vi "Read Field.vi"(7 "field name":string, 8 "error in (no error)":errorcluster, 9 "type code":T1, 10 "value":variant, 11 "Value in":refnum<class "Value.lvclass">) -> (0 "error out":errorcluster, 2 "value out":variant, 3 "Value out":refnum<class "Value.lvclass">)   [LabVIEW 2020, in "Value.lvlib" / "Value.lvclass"]
uses:
  Value.lvclass
  <vilib>/ErrorRing/Error Ring.xnode
  3e63842f-1b42-44b7-bfbc-53574ae558bd.vi
  0df52538-0c37-4fc1-a2a6-aa64d23bd73e.vi
  ea7cb730-9445-4e63-a674-7488b051f0a2.vi
  ecc6d044-d1d6-4258-b554-93b542f000c4.vi
  f0dd0353-13dc-4229-be36-72f5216b3ba3.vi
  663b7534-5be4-4c26-8693-775dffd107bf.vi
  6d95b702-a3d4-47fa-b99c-6e9c691d9abd.vi
  334379f0-c2c1-4fd4-b37a-a75153a3c3c1.vi
  22215a59-2fe5-468e-8a76-07a567f1422d.vi
  3b673ad6-c2bb-415d-ac32-dac8d0585a62.vi
  4907590c-51dd-452d-854a-3f23d6337043.vi
  91e94b60-106e-4a8f-bb72-5d9817169e6a.vi
  c7390ac7-e1e0-4f30-b90a-9159575d946d.vi
  aaf6655d-cd8e-45f8-b77e-a22837ed21e0.vi
  830d96f2-0dcb-4e12-99cb-9e6dde05f73e.vi
  77dc8c9c-6059-4e17-8748-14fb7ec0ac2f.vi
  a9875d30-4bd9-4a8c-a52c-f68dec12aa6b.vi
  6dbc08b8-92b8-4054-99f1-d97896c52856.vi
  c55a9e90-05cb-4a8a-8098-6274f5663967.vi
  316c9c8d-b543-4ebf-942d-59175514938d.vi
  229b0493-3b28-4ef3-8240-f1556a969e00.vi
  76e9d66a-8186-463b-a0b5-702645c41f9e.vi
  c324c6c0-264f-44f1-9003-e2f03347ce10.vi
  99229403-bf4d-41b1-8e34-2119cf99b534.vi
  94649a53-8ca4-4095-9f16-4726c07ca332.vi
  d57c28cb-9096-4c65-b10b-a5dea6344eea.vi
  a983453c-48a8-483e-9635-4b6015360bbf.vi
  3184ba56-7df3-4453-b731-c59013ebea68.vi
  6054442b-7a6b-42bc-83b9-383781339b04.vi
  6affac03-527b-4ec4-b0fc-9a513264455a.vi
  a9131e02-a07e-4dd8-b605-98a98183cd4d.vi
  df721e5c-d840-4c3d-88a1-754951405b27.vi
  37bd5290-b6b7-48eb-a0fa-e2d498b26fe2.vi
  1f354738-e960-4e7d-8bfb-2b975031cf57.vi
  eb45627c-0224-4171-a2ca-7d038fcf7cb5.vi
  763b9c78-21ee-42ab-85a7-a612ad3e0854.vi
  b475763c-3eeb-44d5-9789-6e92f77c8c05.vi
  7e13b756-e5dd-4f30-8145-3e48ab5751a0.vi
  311b836b-25cf-44d6-867a-da423852ab29.vi
  884a57a7-1cc5-4241-a283-3421418f3c32.vi
  e5b34253-12a8-4f36-ae48-ef8a9a19dc9f.vi
  9a6462e7-f1a7-4896-b94c-43e163632ccd.vi
  919939b4-f74b-49d6-a078-a721f5adc92b.vi
  7b5734c8-9551-4087-a43c-2e9c6be36d77.vi
  e7c0ed72-c8d2-4a6e-8d95-57b650344be6.vi
  78a636ab-c8c7-43d5-9c2f-ed25fd418a22.vi
  3f976d8e-f489-4d6c-8102-c644feb36fb3.vi
  2b071918-53f3-414b-a359-069b1376627a.vi
  60c7cc55-0a77-42d8-819b-5811e97bdf1a.vi
  <vilib>/Utility/error.llb/Error Cluster From Error Code.vi
  Type Code.ctl
  Value.lvlib
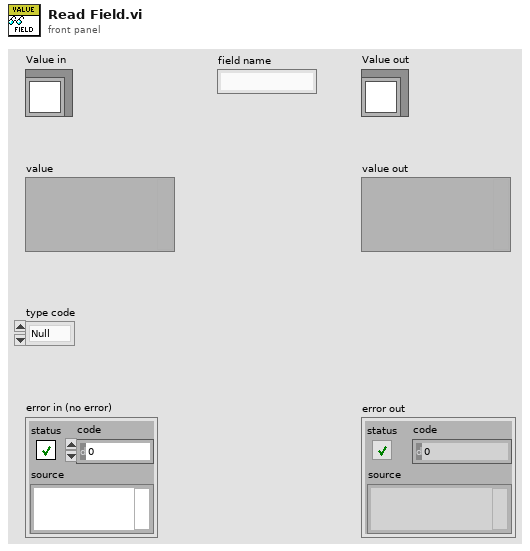
[diagram p1: front panel]
types:
  T1 = typedef "Value.lvlib/Type Code.ctl" = enum8{"Null", "Bool", "BoolA", "Int8", "Int8A", "Int16", "Int16A", "Int32", "Int32A", "Int64", "Int64A", "UInt8", "UInt8A", "UInt16", "UInt16A", "UInt32", "UInt32A", "UInt64", "UInt64A", "Float32", "Float32A", "Float64", "Float64A", "String", "StringA", "Struct", "StructA", "Union", "UnionA", "Any", "AnyA"}
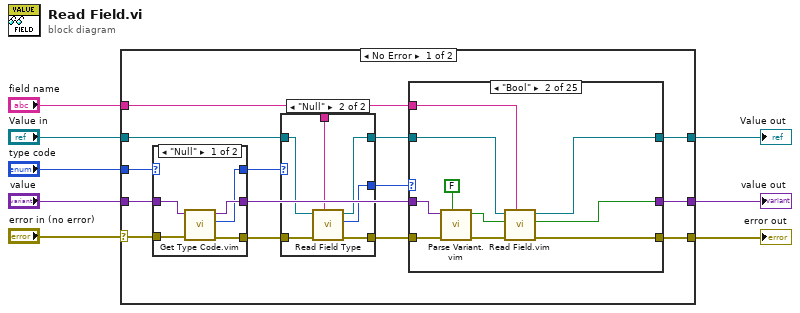
[diagram p0: block diagram]
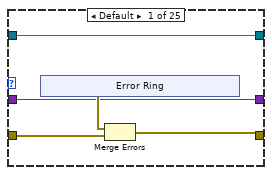
[diagram p4: hidden frame]
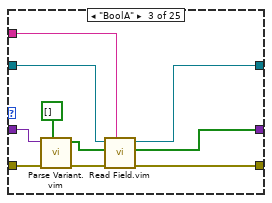
[diagram p5: hidden frame]
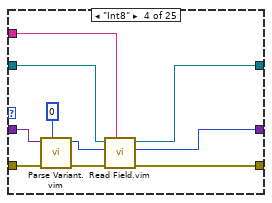
[diagram p6: hidden frame]
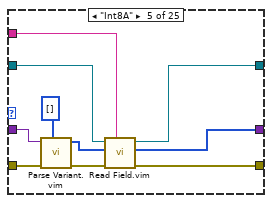
[diagram p7: hidden frame]
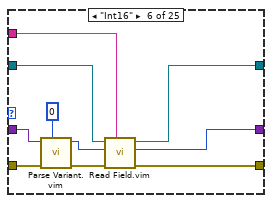
[diagram p8: hidden frame]
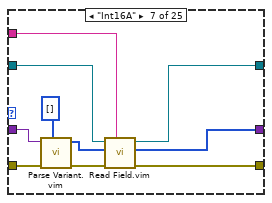
[diagram p9: hidden frame]
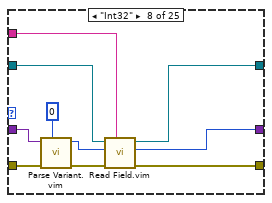
[diagram p10: hidden frame]
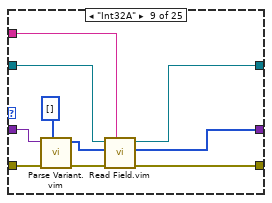
[diagram p11: hidden frame]
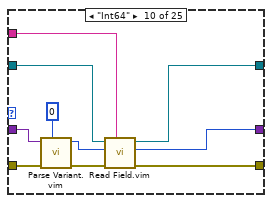
[diagram p12: hidden frame]
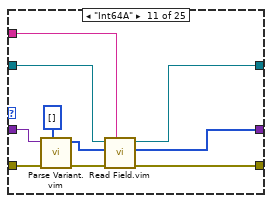
[diagram p13: hidden frame]
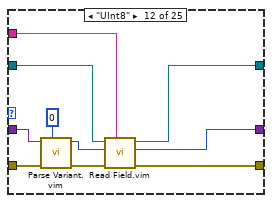
[diagram p14: hidden frame]
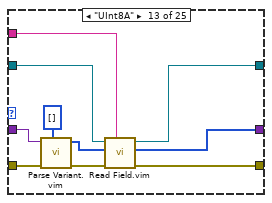
[diagram p15: hidden frame]
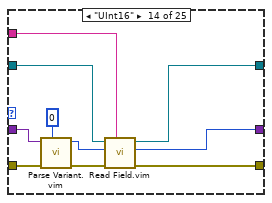
[diagram p16: hidden frame]
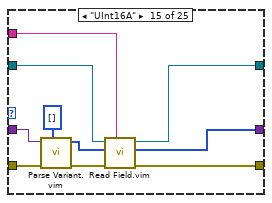
[diagram p17: hidden frame]
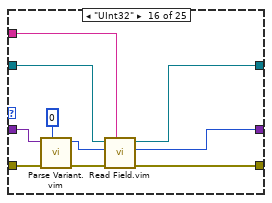
[diagram p18: hidden frame]
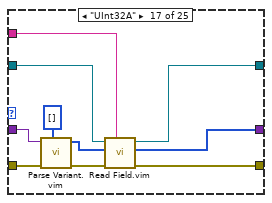
[diagram p19: hidden frame]
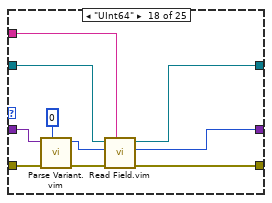
[diagram p20: hidden frame]
diagram:
  n1 = case shown="No Error" "error in (no error)" {
    selector: "error in (no error)" -> [w20 w291]
    tunnel: [w22 w291] -> w7
    tunnel: "Value in" -> [w14 w290]
    tunnel: [w21 w290] -> w5
    tunnel: "field name" -> [w10 _]
    tunnel: "value" -> [w19 w289]
    tunnel: "type code" -> [w17 _]
    tunnel: [w9 w289] -> w1
    frame No Error {
      n2 = case shown="\"Null\"" w17 {
        selector: w17 -> [_ w39]
        tunnel: w20 -> [w36 w38]
        tunnel: [w35 w38] -> w16
        tunnel: w19 -> [w34 w37]
        tunnel: [w33 w37] -> w18
        tunnel: [w32 w39] -> w12
        frame "Null" {
          n3 = call "Get Type Code.vim"("error in"=w36, "default"=w34) -> ("error out"=w35:errorcluster, "type code"=w32:T1, "value"=w33:variant)  [unwired: 7 in]
        }
        frame Default {
        }
      }
      n4 = case shown="\"Null\"" w12 {
        selector: w12 -> [w25 _]
        tunnel: w16 -> [w24 w31]
        tunnel: [w24 w30] -> w15
        tunnel: w14 -> [w23 w29]
        tunnel: [w23 w28] -> w13
        tunnel: w10 -> [_ w27]
        tunnel: [w25 w26] -> w11
        frame Default {
        }
        frame "Null" {
          n5 = call "Read Field Type.vi"("field name"=w27, "error in (no error)"=w31, "Value in"=w29) -> ("error out"=w30:errorcluster, "type code"=w26:T1, "Value out"=w28:refnum<class "Value.lvclass">)  [unwired: 6 in]
        }
      }
      n6 = case shown="\"Bool\"" w11 {
        tunnel: [w43 w55 w66 w76 w86 w96 w106 w116 w126 w136 w147 w156 w166 w176 w186 w196 w206 w216 w226 w236 w246 w256 w266 w276 w286] -> w22
        tunnel: w15 -> [w44 w58 w68 w78 w88 w98 w108 w118 w128 w138 w148 w158 w168 w178 w188 w198 w208 w218 w228 w238 w248 w258 w268 w278 w288]
        tunnel: [w41 w53 w64 w75 w84 w94 w104 w114 w124 w134 w145 w154 w164 w175 w184 w194 w205 w214 w224 w234 w244 w254 w264 w274 w284] -> w21
        tunnel: [w40 w52 w62 w73 w82 w92 w102 w112 w122 w132 w143 w152 w162 w173 w182 w192 w203 w212 w222 w232 w242 w252 w262 w272 w282] -> w9
        tunnel: w13 -> [w41 w51 w61 w72 w81 w91 w101 w111 w121 w131 w141 w151 w161 w172 w181 w191 w202 w211 w221 w231 w241 w251 w261 w271 w281]
        tunnel: w10 -> [_ w50 w60 w70 w80 w90 w100 w110 w120 w130 w140 w150 w160 w170 w180 w190 w200 w210 w220 w230 w240 w250 w260 w270 w280]
        tunnel: w18 -> [w40 w49 w59 w69 w79 w89 w99 w109 w119 w129 w139 w149 w159 w169 w179 w189 w199 w209 w219 w229 w239 w249 w259 w269 w279]
        frame Default {
          n7 = xnode "Error Ring"() -> ("error out"=w42:errorcluster)
          n8 = Merge Errors(w42, w44) -> (w43:errorcluster)
        }
        frame "Bool" {
          n9 = call "Parse Variant.vim"("default"=FALSE, "error in (no error)"=w58, "value"=w49) -> ("error out"=w56:errorcluster, "value out"=w54:bool)  [unwired: 7 in]
          n10 = call "Read Field.vim"("field name"=w50, "error in"=w56, "default"=w54, "Value in"=w51) -> ("error out"=w55:errorcluster, "value"=w52:bool, "Value out"=w53:refnum<class "Value.lvclass">)  [unwired: 5 in]
        }
        frame "BoolA" {
          n11 = call "Parse Variant.vim"("default"=bool[] [], "error in (no error)"=w68, "value"=w59) -> ("error out"=w67:errorcluster, "value out"=w65:bool[])  [unwired: 7 in]
          n12 = call "Read Field.vim"("field name"=w60, "error in"=w67, "default"=w65, "Value in"=w61) -> ("error out"=w66:errorcluster, "value"=w62:bool[], "Value out"=w64:refnum<class "Value.lvclass">)  [unwired: 5 in]
        }
        frame "Int8" {
          n13 = call "Parse Variant.vim"("default"=i8 0, "error in (no error)"=w78, "value"=w69) -> ("error out"=w77:errorcluster, "value out"=w71:i8)  [unwired: 7 in]
          n14 = call "Read Field.vim"("field name"=w70, "error in"=w77, "default"=w71, "Value in"=w72) -> ("error out"=w76:errorcluster, "value"=w73:i8, "Value out"=w75:refnum<class "Value.lvclass">)  [unwired: 5 in]
        }
        frame "Int8A" {
          n15 = call "Parse Variant.vim"("default"=i8[] [], "error in (no error)"=w88, "value"=w79) -> ("error out"=w87:errorcluster, "value out"=w85:i8[])  [unwired: 7 in]
          n16 = call "Read Field.vim"("field name"=w80, "error in"=w87, "default"=w85, "Value in"=w81) -> ("error out"=w86:errorcluster, "value"=w82:i8[], "Value out"=w84:refnum<class "Value.lvclass">)  [unwired: 5 in]
        }
        frame "Int16" {
          n17 = call "Parse Variant.vim"("default"=i16 0, "error in (no error)"=w98, "value"=w89) -> ("error out"=w97:errorcluster, "value out"=w95:i16)  [unwired: 7 in]
          n18 = call "Read Field.vim"("field name"=w90, "error in"=w97, "default"=w95, "Value in"=w91) -> ("error out"=w96:errorcluster, "value"=w92:i16, "Value out"=w94:refnum<class "Value.lvclass">)  [unwired: 5 in]
        }
        frame "Int16A" {
          n19 = call "Parse Variant.vim"("default"=i16[] [], "error in (no error)"=w108, "value"=w99) -> ("error out"=w107:errorcluster, "value out"=w105:i16[])  [unwired: 7 in]
          n20 = call "Read Field.vim"("field name"=w100, "error in"=w107, "default"=w105, "Value in"=w101) -> ("error out"=w106:errorcluster, "value"=w102:i16[], "Value out"=w104:refnum<class "Value.lvclass">)  [unwired: 5 in]
        }
        frame "Int32" {
          n21 = call "Parse Variant.vim"("default"=0, "error in (no error)"=w118, "value"=w109) -> ("error out"=w117:errorcluster, "value out"=w115:i32)  [unwired: 7 in]
          n22 = call "Read Field.vim"("field name"=w110, "error in"=w117, "default"=w115, "Value in"=w111) -> ("error out"=w116:errorcluster, "value"=w112:i32, "Value out"=w114:refnum<class "Value.lvclass">)  [unwired: 5 in]
        }
        frame "Int32A" {
          n23 = call "Parse Variant.vim"("default"=i32[] [], "error in (no error)"=w128, "value"=w119) -> ("error out"=w127:errorcluster, "value out"=w125:i32[])  [unwired: 7 in]
          n24 = call "Read Field.vim"("field name"=w120, "error in"=w127, "default"=w125, "Value in"=w121) -> ("error out"=w126:errorcluster, "value"=w122:i32[], "Value out"=w124:refnum<class "Value.lvclass">)  [unwired: 5 in]
        }
        frame "Int64" {
          n25 = call "Parse Variant.vim"("default"=i64 0, "error in (no error)"=w138, "value"=w129) -> ("error out"=w137:errorcluster, "value out"=w135:i64)  [unwired: 7 in]
          n26 = call "Read Field.vim"("field name"=w130, "error in"=w137, "default"=w135, "Value in"=w131) -> ("error out"=w136:errorcluster, "value"=w132:i64, "Value out"=w134:refnum<class "Value.lvclass">)  [unwired: 5 in]
        }
        frame "Int64A" {
          n27 = call "Parse Variant.vim"("default"=i64[] [], "error in (no error)"=w148, "value"=w139) -> ("error out"=w142:errorcluster, "value out"=w146:i64[])  [unwired: 7 in]
          n28 = call "Read Field.vim"("field name"=w140, "error in"=w142, "default"=w146, "Value in"=w141) -> ("error out"=w147:errorcluster, "value"=w143:i64[], "Value out"=w145:refnum<class "Value.lvclass">)  [unwired: 5 in]
        }
        frame "UInt8" {
          n29 = call "Parse Variant.vim"("default"=u8 0, "error in (no error)"=w158, "value"=w149) -> ("error out"=w157:errorcluster, "value out"=w155:u8)  [unwired: 7 in]
          n30 = call "Read Field.vim"("field name"=w150, "error in"=w157, "default"=w155, "Value in"=w151) -> ("error out"=w156:errorcluster, "value"=w152:u8, "Value out"=w154:refnum<class "Value.lvclass">)  [unwired: 5 in]
        }
        frame "UInt8A" {
          n31 = call "Parse Variant.vim"("default"=u8[] [], "error in (no error)"=w168, "value"=w159) -> ("error out"=w167:errorcluster, "value out"=w165:u8[])  [unwired: 7 in]
          n32 = call "Read Field.vim"("field name"=w160, "error in"=w167, "default"=w165, "Value in"=w161) -> ("error out"=w166:errorcluster, "value"=w162:u8[], "Value out"=w164:refnum<class "Value.lvclass">)  [unwired: 5 in]
        }
        frame "UInt16" {
          n33 = call "Parse Variant.vim"("default"=u16 0, "error in (no error)"=w178, "value"=w169) -> ("error out"=w177:errorcluster, "value out"=w171:u16)  [unwired: 7 in]
          n34 = call "Read Field.vim"("field name"=w170, "error in"=w177, "default"=w171, "Value in"=w172) -> ("error out"=w176:errorcluster, "value"=w173:u16, "Value out"=w175:refnum<class "Value.lvclass">)  [unwired: 5 in]
        }
        frame "UInt16A" {
          n35 = call "Parse Variant.vim"("default"=u16[] [], "error in (no error)"=w188, "value"=w179) -> ("error out"=w187:errorcluster, "value out"=w185:u16[])  [unwired: 7 in]
          n36 = call "Read Field.vim"("field name"=w180, "error in"=w187, "default"=w185, "Value in"=w181) -> ("error out"=w186:errorcluster, "value"=w182:u16[], "Value out"=w184:refnum<class "Value.lvclass">)  [unwired: 5 in]
        }
        frame "UInt32" {
          n37 = call "Parse Variant.vim"("default"=u32 0, "error in (no error)"=w198, "value"=w189) -> ("error out"=w197:errorcluster, "value out"=w195:u32)  [unwired: 7 in]
          n38 = call "Read Field.vim"("field name"=w190, "error in"=w197, "default"=w195, "Value in"=w191) -> ("error out"=w196:errorcluster, "value"=w192:u32, "Value out"=w194:refnum<class "Value.lvclass">)  [unwired: 5 in]
        }
        frame "UInt32A" {
          n39 = call "Parse Variant.vim"("default"=u32[] [], "error in (no error)"=w208, "value"=w199) -> ("error out"=w207:errorcluster, "value out"=w201:u32[])  [unwired: 7 in]
          n40 = call "Read Field.vim"("field name"=w200, "error in"=w207, "default"=w201, "Value in"=w202) -> ("error out"=w206:errorcluster, "value"=w203:u32[], "Value out"=w205:refnum<class "Value.lvclass">)  [unwired: 5 in]
        }
        frame "UInt64" {
          n41 = call "Parse Variant.vim"("default"=u64 0, "error in (no error)"=w218, "value"=w209) -> ("error out"=w217:errorcluster, "value out"=w215:u64)  [unwired: 7 in]
          n42 = call "Read Field.vim"("field name"=w210, "error in"=w217, "default"=w215, "Value in"=w211) -> ("error out"=w216:errorcluster, "value"=w212:u64, "Value out"=w214:refnum<class "Value.lvclass">)  [unwired: 5 in]
        }
        frame "UInt64A" {
          n43 = call "Parse Variant.vim"("default"=u64[] [], "error in (no error)"=w228, "value"=w219) -> ("error out"=w227:errorcluster, "value out"=w225:u64[])  [unwired: 7 in]
          n44 = call "Read Field.vim"("field name"=w220, "error in"=w227, "default"=w225, "Value in"=w221) -> ("error out"=w226:errorcluster, "value"=w222:u64[], "Value out"=w224:refnum<class "Value.lvclass">)  [unwired: 5 in]
        }
        frame "Float32" {
          n45 = call "Parse Variant.vim"("default"=sgl 0.0, "error in (no error)"=w238, "value"=w229) -> ("error out"=w237:errorcluster, "value out"=w235:sgl)  [unwired: 7 in]
          n46 = call "Read Field.vim"("field name"=w230, "error in"=w237, "default"=w235, "Value in"=w231) -> ("error out"=w236:errorcluster, "value"=w232:sgl, "Value out"=w234:refnum<class "Value.lvclass">)  [unwired: 5 in]
        }
        frame "Float64" {
          n47 = call "Parse Variant.vim"("default"=0.0, "error in (no error)"=w248, "value"=w239) -> ("error out"=w247:errorcluster, "value out"=w245:dbl)  [unwired: 7 in]
          n48 = call "Read Field.vim"("field name"=w240, "error in"=w247, "default"=w245, "Value in"=w241) -> ("error out"=w246:errorcluster, "value"=w242:dbl, "Value out"=w244:refnum<class "Value.lvclass">)  [unwired: 5 in]
        }
        frame "Float32A" {
          n49 = call "Parse Variant.vim"("default"=sgl[] [], "error in (no error)"=w258, "value"=w249) -> ("error out"=w257:errorcluster, "value out"=w255:sgl[])  [unwired: 7 in]
          n50 = call "Read Field.vim"("field name"=w250, "error in"=w257, "default"=w255, "Value in"=w251) -> ("error out"=w256:errorcluster, "value"=w252:sgl[], "Value out"=w254:refnum<class "Value.lvclass">)  [unwired: 5 in]
        }
        frame "Float64A" {
          n51 = call "Parse Variant.vim"("default"=dbl[] [], "error in (no error)"=w268, "value"=w259) -> ("error out"=w267:errorcluster, "value out"=w265:dbl[])  [unwired: 7 in]
          n52 = call "Read Field.vim"("field name"=w260, "error in"=w267, "default"=w265, "Value in"=w261) -> ("error out"=w266:errorcluster, "value"=w262:dbl[], "Value out"=w264:refnum<class "Value.lvclass">)  [unwired: 5 in]
        }
        frame "String" {
          n53 = call "Parse Variant.vim"("default"="", "error in (no error)"=w278, "value"=w269) -> ("error out"=w277:errorcluster, "value out"=w275:string)  [unwired: 7 in]
          n54 = call "Read Field.vim"("field name"=w270, "error in"=w277, "default"=w275, "Value in"=w271) -> ("error out"=w276:errorcluster, "value"=w272:string, "Value out"=w274:refnum<class "Value.lvclass">)  [unwired: 5 in]
        }
        frame "StringA" {
          n55 = call "Parse Variant.vim"("default"=string[] [], "error in (no error)"=w288, "value"=w279) -> ("error out"=w287:errorcluster, "value out"=w285:string[])  [unwired: 7 in]
          n56 = call "Read Field.vim"("field name"=w280, "error in"=w287, "default"=w285, "Value in"=w281) -> ("error out"=w286:errorcluster, "value"=w282:string[], "Value out"=w284:refnum<class "Value.lvclass">)  [unwired: 5 in]
        }
      }
    }
    frame Error {
    }
  }
  "value out" <- w1
  "error out" <- w7
  "Value out" <- w5
